vi "PagesUI.vi"() -> ()   [LabVIEW 2015, in "Pages.lvclass"]
uses:
  Pages.lvclass
  <vilib>/NI/Configuration Framework/Node/NodeRef.ctl
  <vilib>/NI/Configuration Framework/Node/NISE_CEF_Node.lvclass
  <vilib>/NI/AMC/Message Queue.ctl
  <vilib>/NI/AMC/Message.ctl
  <vilib>/NI/Tools/Keyed Array/KeyedArray.ctl
  <vilib>/NI/Configuration Framework/Node/UserEventRef.ctl
  <vilib>/NI/Configuration Framework/Controls/EventCluster.ctl
  <vilib>/Utility/sysdir.llb/System Directory Type.ctl
  subVI/Global Settings.vi
  Configuration Tool.lvlib
  <vilib>/NI/Tools/Keyed Array/Tools_KeyedArray.lvlib
  <vilib>/NI/AMC/AMC.lvlib
  <vilib>/NI/Configuration Framework/NISE_CEF_TreeControl.lvlib
panel:
  in  "Main UI Tab":enum32{"Pages"}(tab)
  in  "WebBrowser":refnum<k7>(container)
  in  "user event":T1
  in  "main queue":T2
  in  "node ref":T3
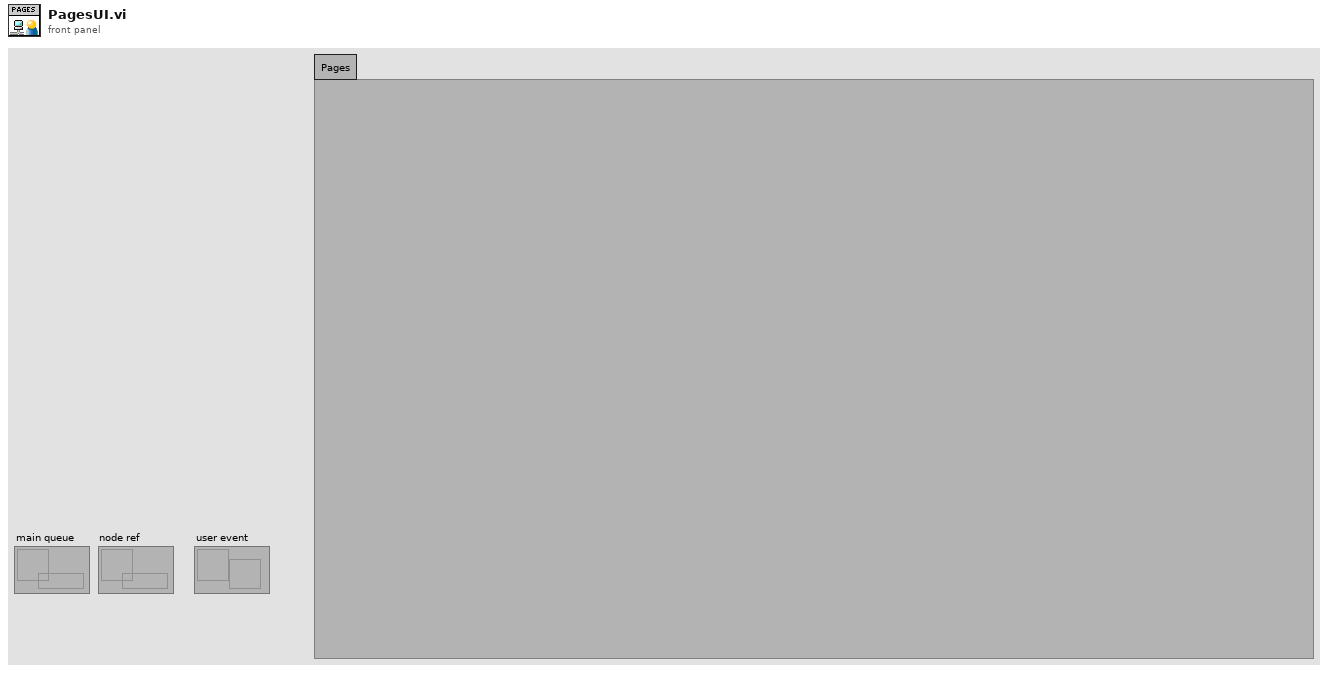
[diagram p1: front panel]
types:
  T1 = typedef "NISE_CEF_Node.lvclass/UserEventRef.ctl" = refnum<user-event>
  T2 = typedef "AMC.lvlib/Message Queue.ctl" = refnum<queue>
  T3 = typedef "NISE_CEF_Node.lvclass/NodeRef.ctl" = refnum<data-value>
  T4 = typedef "System Directory Type.ctl" = i32
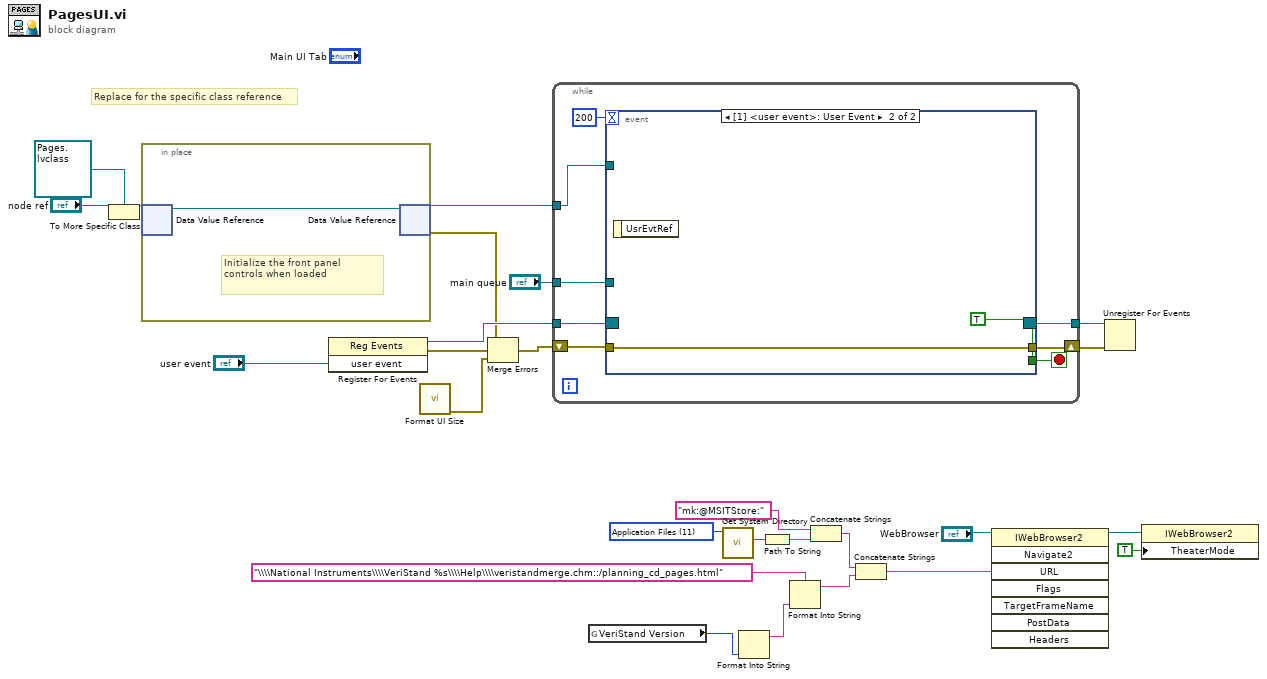
[diagram p0: block diagram]
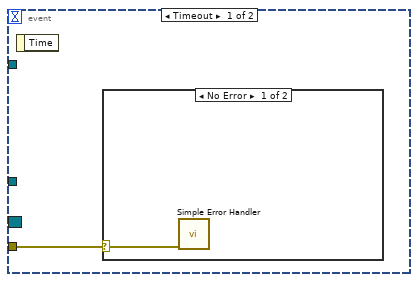
[diagram p2: hidden frame]
diagram:
  w26 = T4 11 items=["User Home"=0, "User Desktop"=1, "User Documents"=2, "User Application Data"=3, "User Preferences"=4, "User Temporary"=5, "Public Documents"=6, "Public Application Data"=7, "Public Preferences"=8, "Public Cache"=13, "System Core Libraries"=9, "System Installed Libraries"=10, "Application Files"=11, "Boot Volume Root"=12] ("system directory type")
  # "Replace for the specific class reference"
  n1 = To More Specific Class(target class=refnum<data-value> refnum ("data value reference"), reference="node ref") -> (specific class reference=w10:refnum<data-value>)  [unwired: 1 in, 1 out]
  n2 = in-place {
    # "Initialize the front panel controls when loaded"
    n3 = in-place-dvr #1(w10) -> (w27:refnum<class "Pages.lvclass">)  [unwired: 1 out]
    n4 = in-place-dvr #1(w27) -> (w17:refnum<data-value>, w7:errorcluster)
  }
  n5 = register-events("user event") -> (reference out=w14:refnum<event-registration>, error out=w8:errorcluster)  [unwired: 2 in]
  n6 = call "Format UI Size.vi"() -> ("error out"=w3:errorcluster)  [unwired: 11 in]
  n7 = Merge Errors(w7, w8, w3) -> (w6:errorcluster)
  n8 = while {
    tunnel: w17 -> [w35]
    tunnel: "main queue" -> [w34]
    tunnel: w14 -> [w32]
    tunnel: [w31] -> w13
    shift-right: [w29] -> w12
    shift-left: w6 -> [w28]
    stop <- w30 stop-if-true
    n9 = event shown="[1] <user event>: User Event" {
      selector: w32 -> [_ _]
      dyn-events: [_ _] -> w31
      timeout: 200 -> [_ _]
      tunnel: w35 -> [_ _]
      tunnel: w34 -> [_ _]
      tunnel: [_ TRUE] -> w30
      tunnel: [_ w38] -> w29
      tunnel: w28 -> [w36 w38]
      event Timeout {
        n10 = event-data() -> ()  [unwired: 1 in, 1 out]
        n11 = case shown="No Error" w36 {
          selector: w36 -> [w37 _]
          frame No Error {
            n12 = call <vilib>:"Simple Error Handler.vi"("error in (no error)"=w37) -> ()  [unwired: 4 in, 5 out]
          }
          frame Error {
          }
        }
      }
      event User Event {
        n13 = event-data() -> ()  [unwired: 1 in, 1 out]
      }
    }
  }
  n14 = global read "Global Settings.vi" "VeriStand Version"() -> (w2:enum16{"2013", "2014", "2015", "2016"})
  n15 = call <vilib>:"Get System Directory.vi"("system directory type"=w26) -> ("system directory"=w25:path)  [unwired: 10 in]
  n16 = Format Into String(w2) -> (resulting string=w1:string)  [unwired: 3 in, 1 out]
  n17 = Path To String(path=w25) -> (string=w24:string)
  n18 = Format Into String(format string="\\\\National Instruments\\\\VeriStand %s\\\\Help\\\\veristandmerge.chm::/planning_cd_pages.html", w1) -> (resulting string=w21:string)  [unwired: 2 in, 1 out]
  n19 = Concatenate Strings("mk:@MSITStore:" ("concatenated string"), w24) -> (w22:string)
  n20 = Concatenate Strings(w22, w21) -> (w19:string)
  n21 = invoke class="IWebBrowser2" method="Navigate2"(reference="WebBrowser", "URL"=w19) -> (reference out=w5:refnum<k7>)  [unwired: 6 in, 7 out]
  n22 = Unregister For Events(event registration refnum=w13, error in=w12) -> ()  [unwired: 1 out]
  n23 = property class="IWebBrowser2"(reference=w5, "TheaterMode"=TRUE) -> ()  [unwired: 1 in, 2 out]
